vi "Get PXI Device List.vi"(7 "Filter Type":T1=enum."Product Name", 8 "error in (no error)":errorcluster, 10 "Filter Names":string[](array[string]), 11 "Target IP Address":string="10.1.128.170") -> (0 "error out":errorcluster, 2 "Alias":string[](array[string]), 3 "Name and Alias":string[](array[string]))   [LabVIEW 2015, in "Resource Management.lvlib"]
uses:
  Resource Management.lvlib
  Types/Filter Type.ctl
  <vilib>/nisyscfg/nisyscfg.lvlib
  <resource>/objmgr/nicriosae.rc
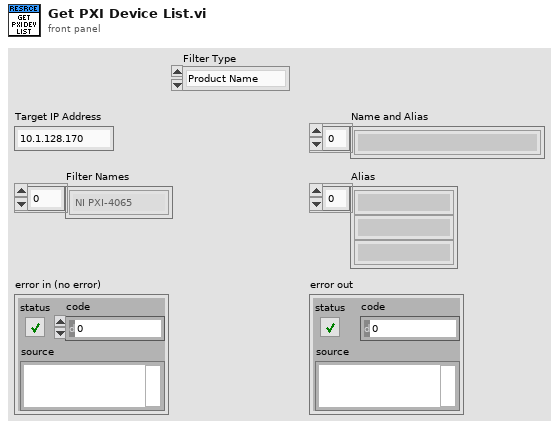
[diagram p1: front panel]
types:
  T1 = typedef "Resource Management.lvlib/Filter Type.ctl" = enum16{"Device Category", "Product Name", "Ethernet", "XNET", "VISA", "FPGA", "EtherCAT Master", "DAQmx"}
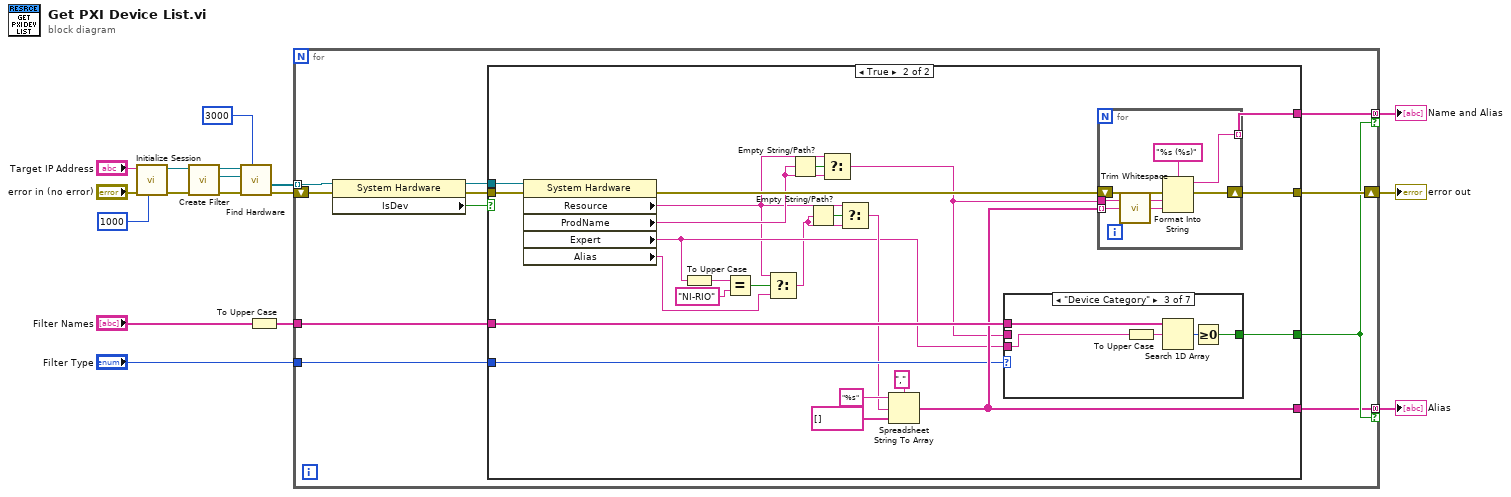
[diagram p0: block diagram]
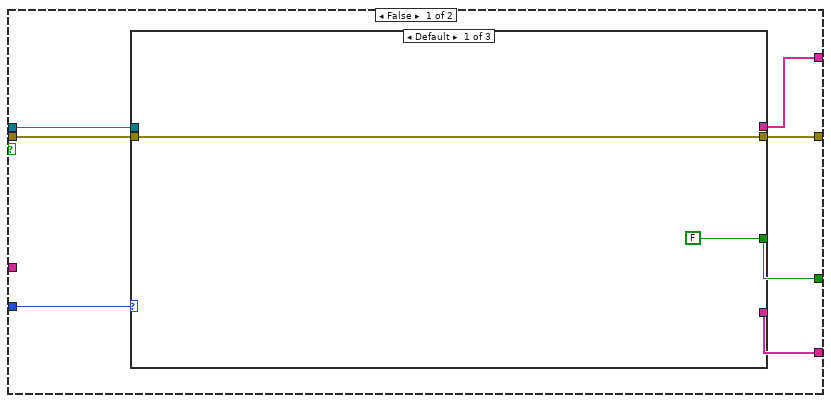
[diagram p2: hidden frame]
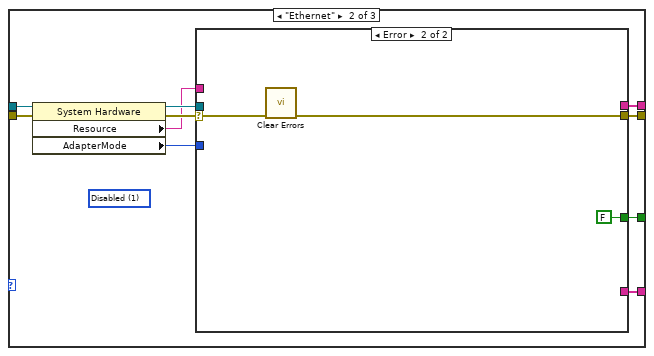
[diagram p3: hidden frame]
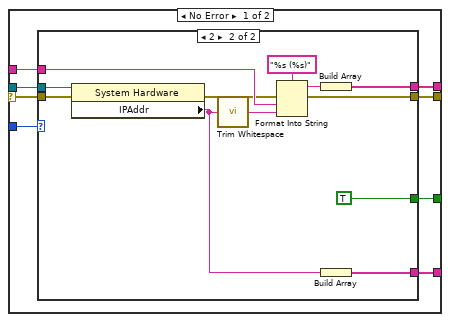
[diagram p4: hidden frame]
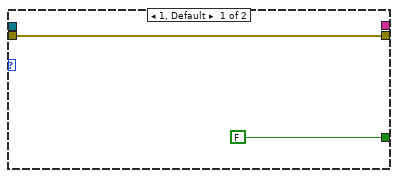
[diagram p5: hidden frame]
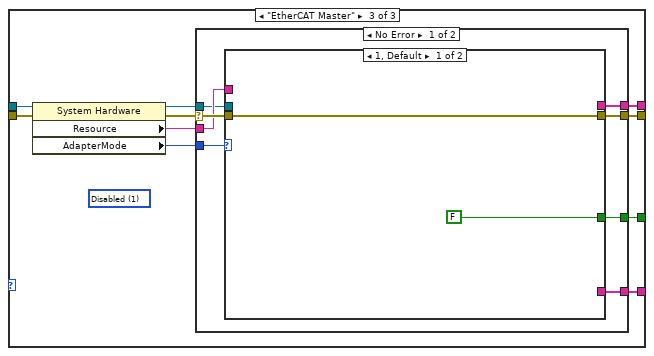
[diagram p6: hidden frame]
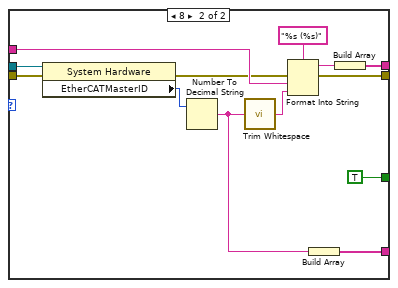
[diagram p7: hidden frame]
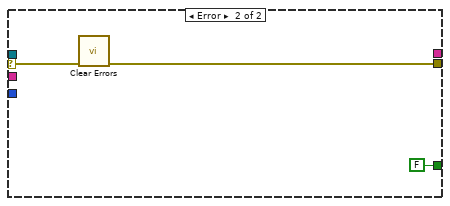
[diagram p8: hidden frame]
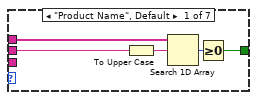
[diagram p9: hidden frame]
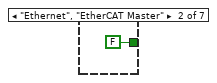
[diagram p10: hidden frame]
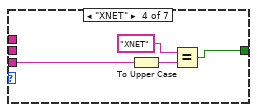
[diagram p11: hidden frame]
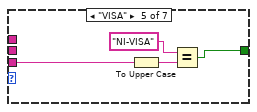
[diagram p12: hidden frame]
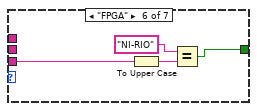
[diagram p13: hidden frame]
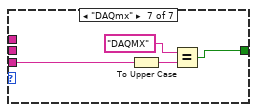
[diagram p14: hidden frame]
diagram:
  n1 = call <vilib>:"Initialize Session.vi"("Connect Timeout (4000 ms)"=u32 1000, "error in (no error)"="error in (no error)", "Target (localhost)"="Target IP Address") -> ("error out"=w9:errorcluster, "Session out"=w7:refnum<k21>)  [unwired: 7 in]
  n2 = call <vilib>:"Create Filter.vi"("error in (no error)"=w9, "Session in"=w7) -> ("error out"=w2:errorcluster, "Filter out"=w1:refnum<k20>, "Session out"=w8:refnum<k21>)  [unwired: 7 in]
  n3 = call <vilib>:"Find Hardware.vi"("Remote Timeout (300,000 ms)"=u32 3000, "error in (no error)"=w2, "Filter in"=w1, "Session in"=w8) -> ("error out"=w11:errorcluster, "Resources out"=w10:refnum<k20>[])  [unwired: 4 in, 2 out]
  n4 = To Upper Case(1:"Filter Names") -> (0:w5:string[])
  n5 = for {
    tunnel: w10 -> [w20] mode=indexing
    tunnel: [w28] -> w13 mode=concatenating if=w25
    shift-right: [w27] -> w14
    shift-left: w11 -> [w22]
    tunnel: [w24] -> w15 mode=concatenating if=w25
    tunnel: w5 -> [w26]
    tunnel: "Filter Type" -> [w23]
    n6 = property class="System Hardware"(reference=w20, error in=w22) -> (reference out=w19:refnum<k20>, error out=w21:errorcluster, "IsDev"=w18:bool)
    n7 = case shown="True" w18 {
      tunnel: [w29 w132] -> w28
      tunnel: [w32 w130] -> w27
      tunnel: w26 -> [_ w129]
      tunnel: [w31 w128] -> w25
      tunnel: [w30 w124] -> w24
      tunnel: w23 -> [w33 w123]
      tunnel: w21 -> [w35 w117]
      tunnel: w19 -> [w34 w116]
      frame False {
        n8 = case shown="Default" w33 {
          tunnel: w35 -> [w37 w47 w82]
          tunnel: w34 -> [_ w46 w81]
          tunnel: [w37 w43 w78] -> w32
          tunnel: [FALSE w42 w77] -> w31
          tunnel: [_ w40 w75] -> w30
          tunnel: [_ w39 w74] -> w29
          frame Default {
          }
          frame "Ethernet" {
            (unwired) u32 1 items=["Disabled"=1, "TCP/IP Ethernet"=2, "Deterministic"=4, "EtherCAT"=8, "TCP/IP WLAN Connect"=32, "TCP/IP WLAN Create"=64] ("Network Adapters:Adapter Mode")
            n9 = property class="System Hardware"(reference=w46, error in=w47) -> (reference out=w41:refnum<k20>, error out=w44:errorcluster, "Resource"=w38:string, "AdapterMode"=w45:u32)
            n10 = case shown="Error" w44 {
              selector: w44 -> [w54 w72]
              tunnel: w45 -> [w55 _]
              tunnel: [w49 w71] -> w43
              tunnel: w38 -> [w53 _]
              tunnel: [w52 FALSE] -> w42
              tunnel: w41 -> [w51 _]
              tunnel: [w50 _] -> w40
              tunnel: [w48 _] -> w39
              frame No Error {
                n11 = case shown="2" w55 {
                  tunnel: w54 -> [w56 w67]
                  tunnel: w53 -> [_ w65]
                  tunnel: [FALSE TRUE] -> w52
                  tunnel: w51 -> [_ w66]
                  tunnel: [_ w58] -> w50
                  tunnel: [w56 w62] -> w49
                  tunnel: [_ w59] -> w48
                  frame 1, Default {
                  }
                  frame 2 {
                    n12 = property class="System Hardware"(reference=w66, error in=w67) -> (error out=w63:errorcluster, "IPAddr"=w64:string)  [unwired: 1 out]
                    n13 = call <vilib>:"Trim Whitespace.vi"("string"=w64) -> ("trimmed string"=w69:string)  [unwired: 1 in]
                    n14 = Format Into String(format string="%s (%s)", error in=w63, w65, w69) -> (resulting string=w60:string, error out=w62:errorcluster)  [unwired: 1 in]
                    n15 = Build Array(w60) -> (w59:string[])
                    n16 = Build Array(w64) -> (w58:string[])
                  }
                }
              }
              frame Error {
                n17 = call <vilib>:"Clear Errors.vi"("error in (no error)"=w72) -> ("error out"=w71:errorcluster)  [unwired: 5 in, 1 out]
              }
            }
          }
          frame "EtherCAT Master" {
            (unwired) u32 1 items=["Disabled"=1, "TCP/IP Ethernet"=2, "Deterministic"=4, "EtherCAT"=8, "TCP/IP WLAN Connect"=32, "TCP/IP WLAN Create"=64] ("Network Adapters:Adapter Mode")
            n18 = property class="System Hardware"(reference=w81, error in=w82) -> (reference out=w76:refnum<k20>, error out=w79:errorcluster, "Resource"=w73:string, "AdapterMode"=w80:u32)
            n19 = case shown="No Error" w79 {
              selector: w79 -> [w89 w108]
              tunnel: w80 -> [w90 _]
              tunnel: [w84 w107] -> w78
              tunnel: w73 -> [w88 _]
              tunnel: [w87 FALSE] -> w77
              tunnel: w76 -> [w86 _]
              tunnel: [w85 _] -> w75
              tunnel: [w83 _] -> w74
              frame No Error {
                n20 = case shown="1, Default" w90 {
                  tunnel: w89 -> [w91 w103]
                  tunnel: w88 -> [_ w101]
                  tunnel: [FALSE TRUE] -> w87
                  tunnel: w86 -> [_ w102]
                  tunnel: [_ w95] -> w85
                  tunnel: [w91 w99] -> w84
                  tunnel: [_ w96] -> w83
                  frame 1, Default {
                  }
                  frame 8 {
                    n21 = property class="System Hardware"(reference=w102, error in=w103) -> (error out=w100:errorcluster, "EtherCATMasterID"=w94:u32)  [unwired: 1 out]
                    n22 = Number To Decimal String(number=w94) -> (decimal integer string=w93:string)  [unwired: 1 in]
                    n23 = call <vilib>:"Trim Whitespace.vi"("string"=w93) -> ("trimmed string"=w105:string)  [unwired: 1 in]
                    n24 = Format Into String(format string="%s (%s)", error in=w100, w101, w105) -> (resulting string=w97:string, error out=w99:errorcluster)  [unwired: 1 in]
                    n25 = Build Array(w93) -> (w95:string[])
                    n26 = Build Array(w97) -> (w96:string[])
                  }
                }
              }
              frame Error {
                n27 = call <vilib>:"Clear Errors.vi"("error in (no error)"=w108) -> ("error out"=w107:errorcluster)  [unwired: 5 in, 1 out]
              }
            }
          }
        }
      }
      frame True {
        n28 = property class="System Hardware"(reference=w116, error in=w117) -> (error out=w131:errorcluster, "Resource"=w111:string, "ProdName"=w118:string, "Expert"=w113:string, "Alias"=w109:string)  [unwired: 1 out]
        n29 = To Upper Case(1:w113) -> (0:w115:string)
        n30 = Equal?(x=w115, y="NI-RIO" ("x")) -> (x = y?=w112:bool)
        n31 = Select(t=w111, s=w112, f=w109) -> (s? t:f=w110:string)
        n32 = Empty String/Path?(string/path=w118) -> (empty?=w122:bool)
        n33 = Empty String/Path?(string/path=w110) -> (empty?=w121:bool)
        n34 = Select(t=w111, s=w122, f=w118) -> (s? t:f=w120:string)
        n35 = Select(t=w111, s=w121, f=w110) -> (s? t:f=w119:string)
        n36 = Spreadsheet String To Array(delimiter (Tab)=",", format string="%s", spreadsheet string=w119, array type (2D Dbl)=string[] []) -> (array=w124:string[])
        n37 = case shown="\"Device Category\"" w123 {
          tunnel: w129 -> [w137 _ w143 _ _ _ _]
          tunnel: w120 -> [w136 _ _ _ _ _ _]
          tunnel: [w134 FALSE w141 w145 w149 w153 w157] -> w128
          tunnel: w113 -> [_ _ w140 w147 w151 w155 w159]
          frame "Product Name", Default {
            n38 = To Upper Case(1:w136) -> (0:w133:string)
            n39 = Search 1D Array(1D array=w137, element=w133) -> (index of element=w135:i32)  [unwired: 1 in]
            n40 = Greater Or Equal To 0?(x=w135) -> (x >= 0?=w134:bool)
          }
          frame "Ethernet", "EtherCAT Master" {
          }
          frame "Device Category" {
            n41 = To Upper Case(1:w140) -> (0:w139:string)
            n42 = Search 1D Array(1D array=w143, element=w139) -> (index of element=w142:i32)  [unwired: 1 in]
            n43 = Greater Or Equal To 0?(x=w142) -> (x >= 0?=w141:bool)
          }
          frame "XNET" {
            n44 = To Upper Case(1:w147) -> (0:w146:string)
            n45 = Equal?(x="XNET", y=w146) -> (x = y?=w145:bool)
          }
          frame "VISA" {
            n46 = To Upper Case(1:w151) -> (0:w150:string)
            n47 = Equal?(x="NI-VISA", y=w150) -> (x = y?=w149:bool)
          }
          frame "FPGA" {
            n48 = To Upper Case(1:w155) -> (0:w154:string)
            n49 = Equal?(x="NI-RIO", y=w154) -> (x = y?=w153:bool)
          }
          frame "DAQmx" {
            n50 = To Upper Case(1:w159) -> (0:w158:string)
            n51 = Equal?(x="DAQMX" ("Display"), y=w158) -> (x = y?=w157:bool)
          }
        }
        n52 = for {
          tunnel: w120 -> [w163]
          tunnel: w124 -> [w161] mode=indexing
          shift-right: [w164] -> w130
          shift-left: w131 -> [w165]
          tunnel: [w166] -> w132 mode=indexing
          n53 = call <vilib>:"Trim Whitespace.vi"("string"=w161) -> ("trimmed string"=w162:string)  [unwired: 1 in]
          n54 = Format Into String(format string="%s (%s)", error in=w165, w163, w162) -> (resulting string=w166:string, error out=w164:errorcluster)  [unwired: 1 in]
        }
      }
    }
  }
  "Name and Alias" <- w13
  "Alias" <- w15
  "error out" <- w14
